vi "Flash Dummy.vi"(8 "Error In":errorcluster) -> (0 "Error Out":errorcluster)   [LabVIEW 2023]
doc: "This VI only shows and hides its own front panel. This is used in some scripting situations to cause the scripted diagram to regain focus so selected objects obtain marching ants."
panel:
  # "Window will run transparently so it should not show up and actually flash."
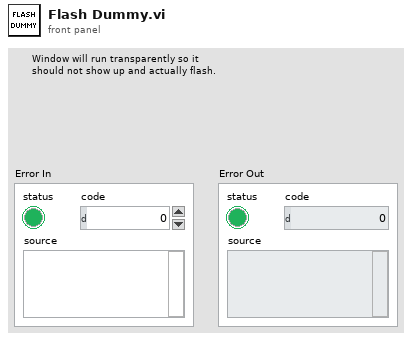
[diagram p1: front panel]
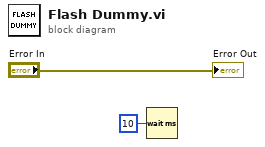
[diagram p0: block diagram]
diagram:
  n1 = Wait (ms)(milliseconds to wait=u32 10) -> ()  [unwired: 1 out]
  "Error Out" <- "Error In"
